vi "外观 1.vi"(0 "Data In":T5 caption="数据输入", 2 "Display State In":T3 caption="显示状态输入", 3 "Container State":T4 caption="容器状态") -> (6 "Data Out":T5 caption="数据输出", 7 "Display State Out":T3 caption="显示状态输出", 8 "Action":T2 caption="动作")   [LabVIEW 2016, in "曲线模型.xctl"]
uses:
  <vilib>/_xctls/Container State.ctl
  <vilib>/_xctls/Action.ctl
  <vilib>/_xctls/XControlSupport.lvlib
  <vilib>/Utility/config.llb/NI_LVConfig.lvlib
panel:
  in  "曲线模型":T1={"标液浓度1"=0.0, "样品1 F0"=0.0, "样品1 F1"=0.0, "测量吸光度1"=0.0, "样品1启用"=FALSE, "标液浓度2"=0.0, "样品2 F0"=0.0, "样品2 F1"=0.0, "测量吸光度2"=0.0, "样品2启用"=FALSE, "标液浓度3"=0.0, "样品3 F0"=0.0, "样品3 F1"=0.0, "测量吸光度3"=0.0, "样品3启用"=FALSE, "标液浓度4"=0.0, "样品4 F0"=0.0, "样品4 F1"=0.0, "测量吸光度4"=0.0, "样品4启用"=FALSE, "标液浓度5"=0.0, "样品5 F0"=0.0, "样品5 F1"=0.0, "测量吸光度5"=0.0, "样品5启用"=FALSE, "模型"=enum."线性", "method"=0, "精度"=4.0, "XY图"=[], "拟合公式"="", "r^2"=0.0} {"method" items=["最小二乘", "最小绝对残差", "Bisquare"]; "r^2" format="%.7g"}
  # "标液浓度"
  # "F0"
  # "F1"
  # "吸光值显示"
  # "样品一"
  # "辅\n助\n计\n算\n区"
  # "样品二"
  # "样品三"
  # "样品四"
  # "样品五"
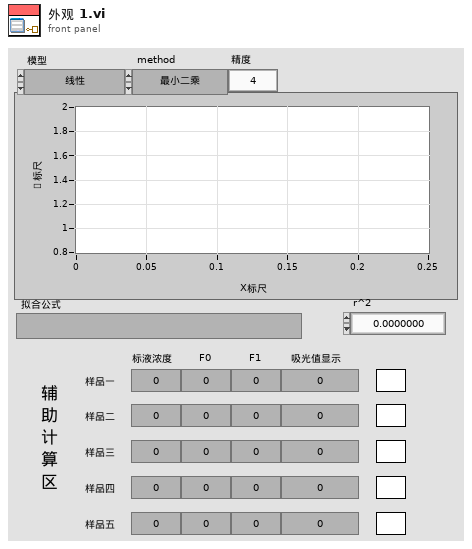
[diagram p1: front panel]
types:
  T1 = typedef "曲线模型.xctl/曲线模型外观.ctl" = cluster{"标液浓度1":dbl, "样品1 F0":dbl, "样品1 F1":dbl, "测量吸光度1":dbl, "样品1启用":bool, "标液浓度2":dbl, "样品2 F0":dbl, "样品2 F1":dbl, "测量吸光度2":dbl, "样品2启用":bool, "标液浓度3":dbl, "样品3 F0":dbl, "样品3 F1":dbl, "测量吸光度3":dbl, "样品3启用":bool, "标液浓度4":dbl, "样品4 F0":dbl, "样品4 F1":dbl, "测量吸光度4":dbl, "样品4启用":bool, "标液浓度5":dbl, "样品5 F0":dbl, "样品5 F1":dbl, "测量吸光度5":dbl, "样品5启用":bool, "模型":enum32{"线性", "多项式"}, "method":u16, "精度":dbl, "XY图":cluster{"X Values":dbl[], "Y Values":dbl[]}[], "拟合公式":string, "r^2":dbl}
  T2 = typedef "XControlSupport.lvlib/Action.ctl" = cluster{"Data Changed?":bool, "State Changed?":bool, "Action Name":string}
  T3 = typedef "曲线模型.xctl/状态 1.ctl" = cluster{"模型选择":cluster{"参数":u8, "测量模式":u8, "量程":u8}}
  T4 = typedef "XControlSupport.lvlib/Container State.ctl" = cluster{"Indicator?":bool, "Run Mode?":bool, " Refnum":refnum<vi>}
  T5 = typedef "曲线模型.xctl/数据 1.ctl" = cluster{"X^2":dbl, "X":dbl, "B":dbl}
  T6 = cluster{"曲线模型":cluster{"标液浓度1":dbl, "样品1 F0":dbl, "样品1 F1":dbl, "测量吸光度1":dbl, "样品1启用":bool, "标液浓度2":dbl, "样品2 F0":dbl, "样品2 F1":dbl, "测量吸光度2":dbl, "样品2启用":bool, "标液浓度3":dbl, "样品3 F0":dbl, "样品3 F1":dbl, "测量吸光度3":dbl, "样品3启用":bool, "标液浓度4":dbl, "样品4 F0":dbl, "样品4 F1":dbl, "测量吸光度4":dbl, "样品4启用":bool, "标液浓度5":dbl, "样品5 F0":dbl, "样品5 F1":dbl, "测量吸光度5":dbl, "样品5启用":bool, "模型":enum32{"线性", "多项式"}, "method":u16, "精度":dbl, "XY图":cluster{"X Values":dbl[], "Y Values":dbl[]}[], "拟合公式":string, "r^2":dbl}, "Polynomial Coefficients":dbl[]}
  T7 = typedef "NI_LVConfig.lvlib/Config Data RefNum.ctl" = refnum<k1>
  T8 = cluster{"Polynomial Coefficients[0]":dbl, "Polynomial Coefficients[1]":dbl, "Polynomial Coefficients[2]":dbl}
  T9 = cluster{"标液浓度1":dbl, "样品1 F0":dbl, "样品1 F1":dbl, "测量吸光度1":dbl, "样品1启用":bool, "标液浓度2":dbl, "样品2 F0":dbl, "样品2 F1":dbl, "测量吸光度2":dbl, "样品2启用":bool, "标液浓度3":dbl, "样品3 F0":dbl, "样品3 F1":dbl, "测量吸光度3":dbl, "样品3启用":bool, "标液浓度4":dbl, "样品4 F0":dbl, "样品4 F1":dbl, "测量吸光度4":dbl, "样品4启用":bool, "标液浓度5":dbl, "样品5 F0":dbl, "样品5 F1":dbl, "测量吸光度5":dbl, "样品5启用":bool, "模型":enum32{"线性", "多项式"}, "method":u16, "精度":dbl, "XY图":cluster{"X Values":dbl[], "Y Values":dbl[]}[], "拟合公式":string, "r^2":dbl}
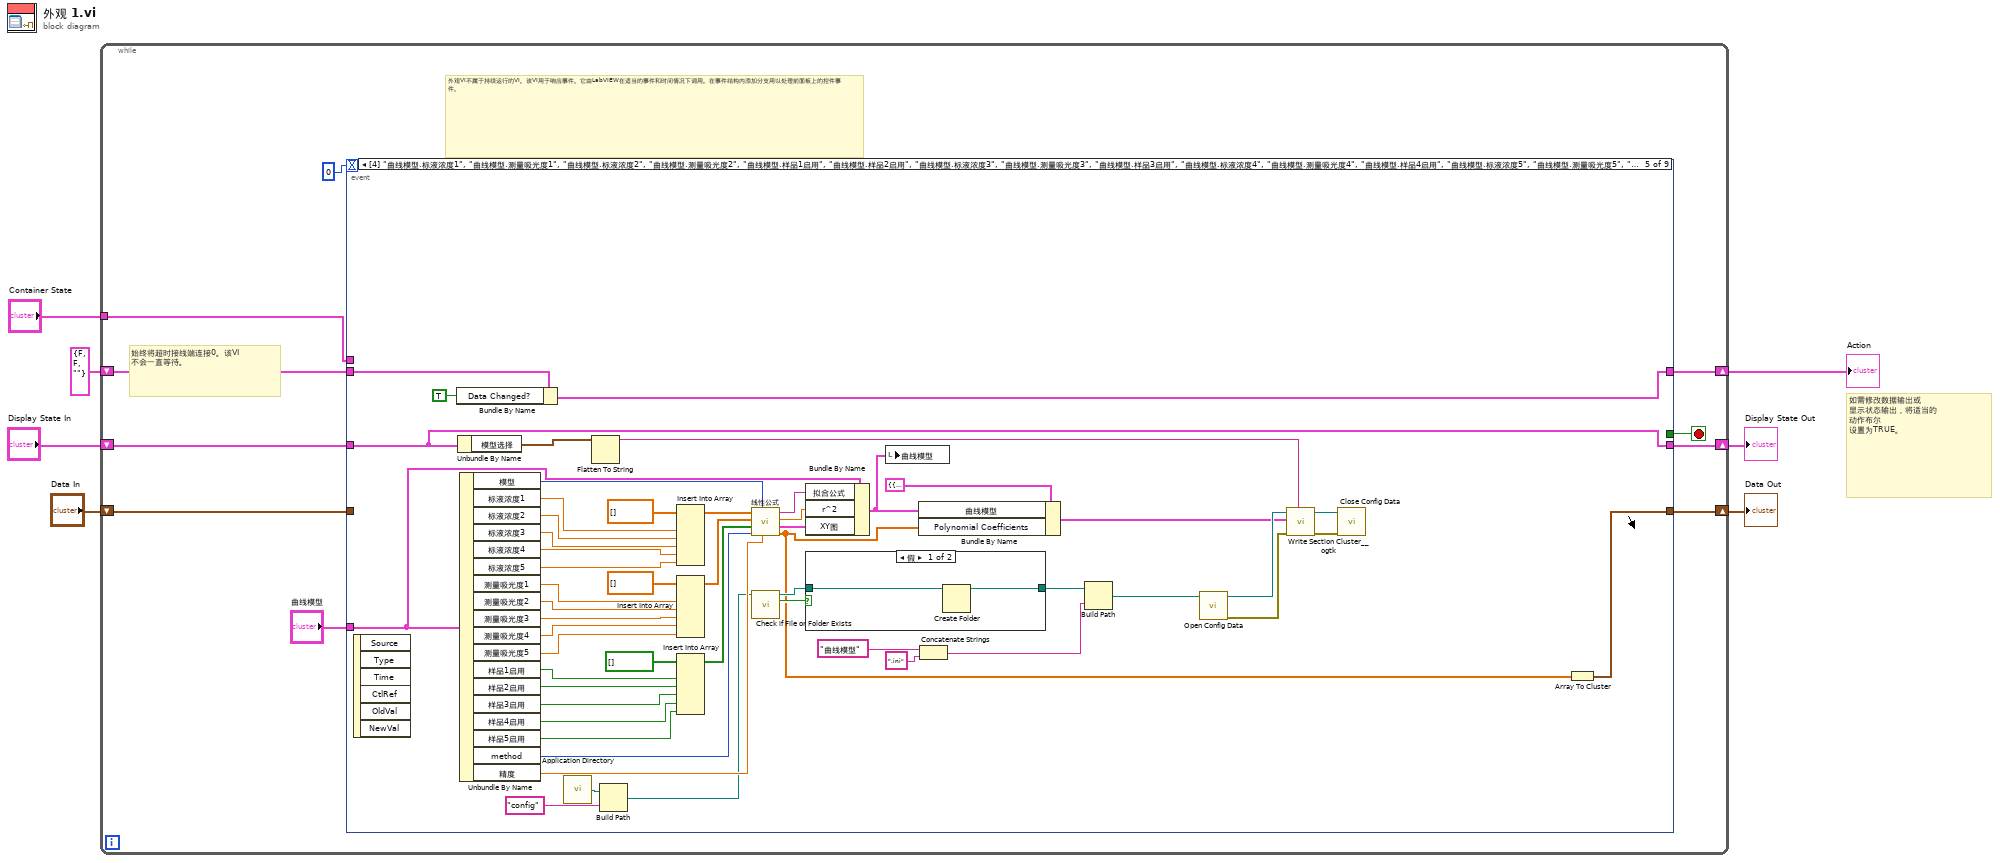
[diagram p0: block diagram]
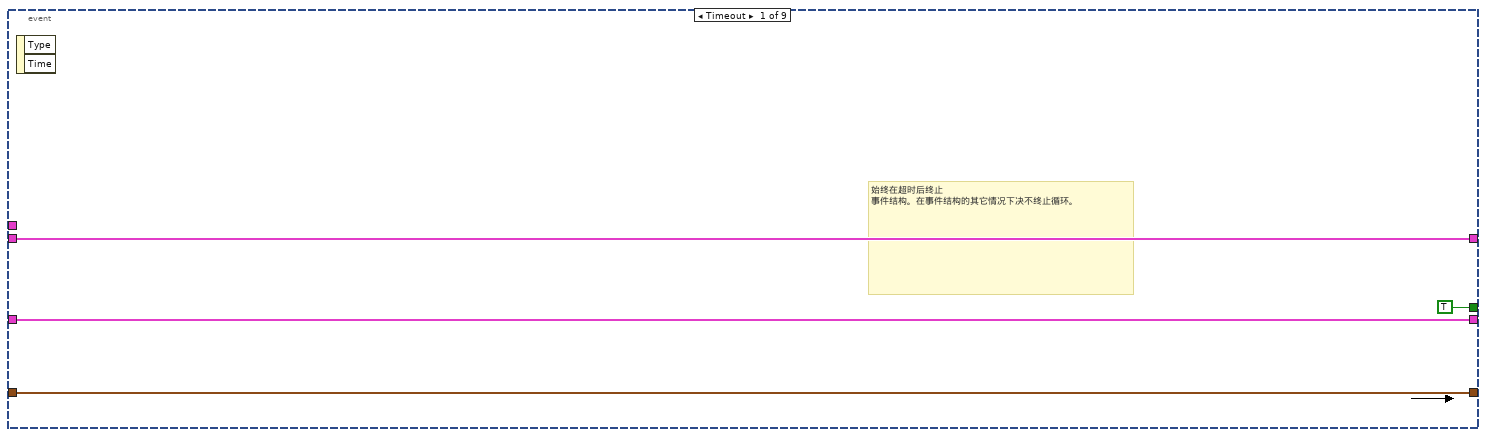
[diagram p2: hidden frame]
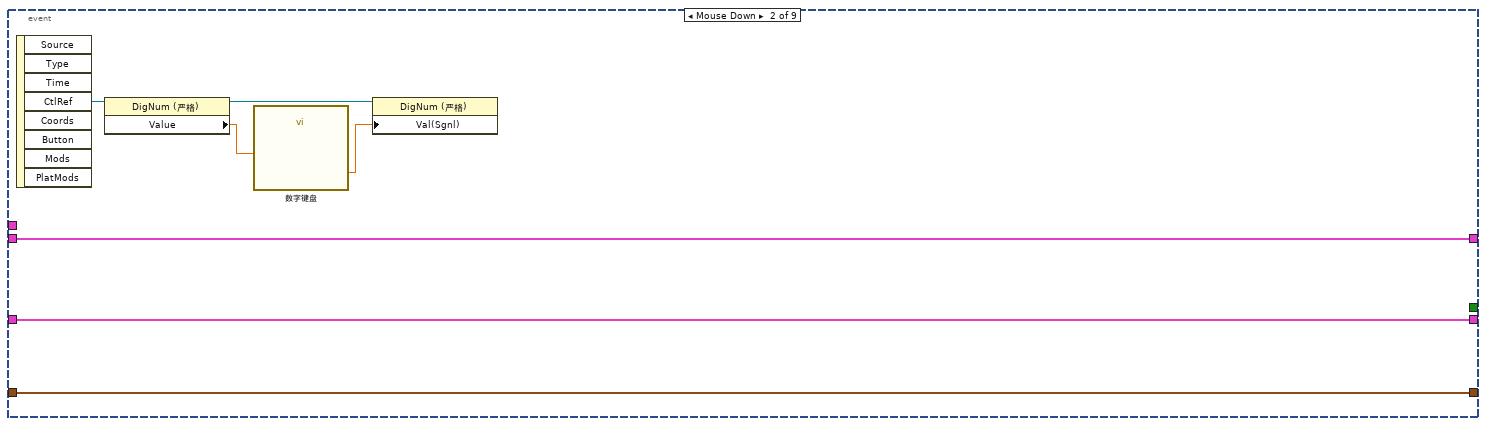
[diagram p3: hidden frame]
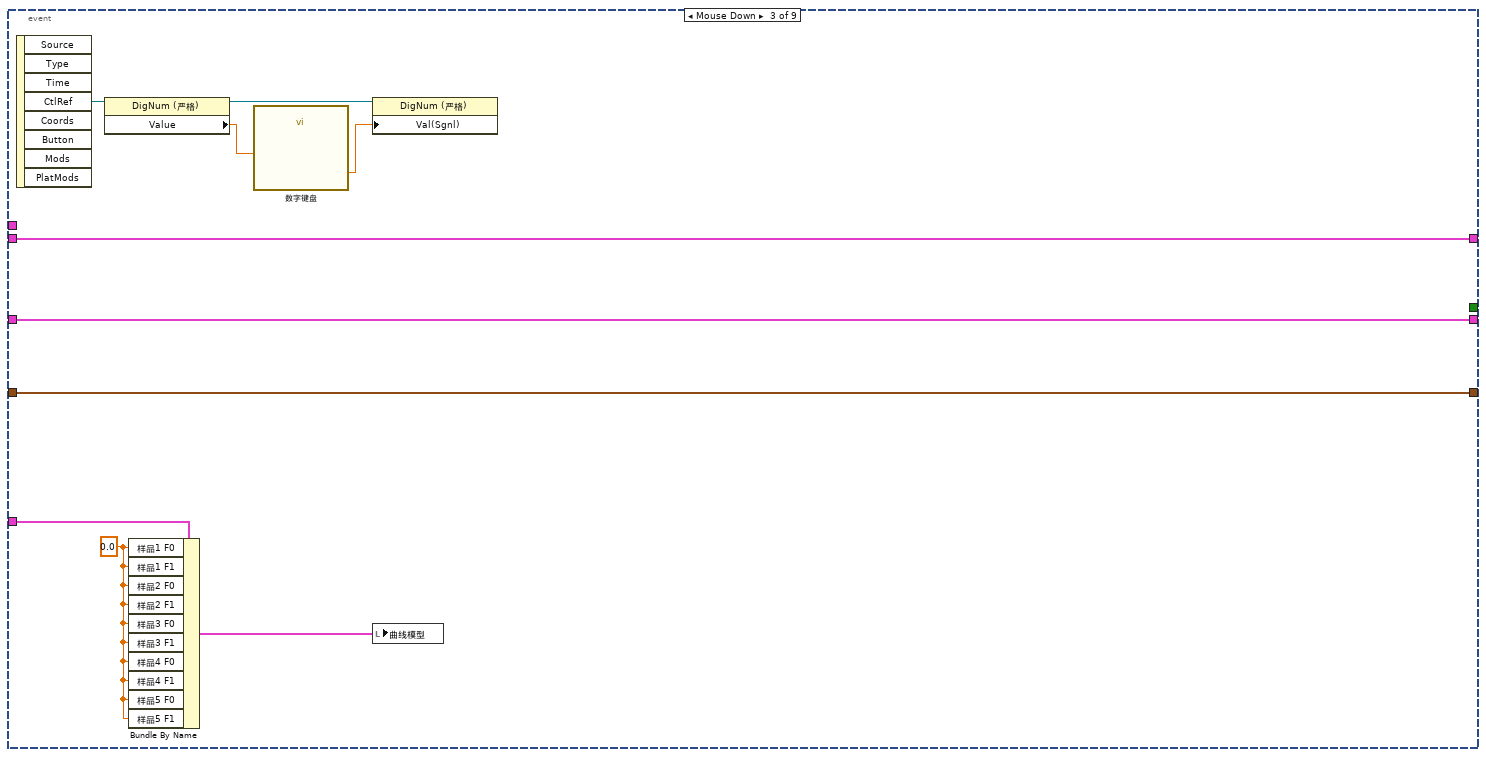
[diagram p4: hidden frame]
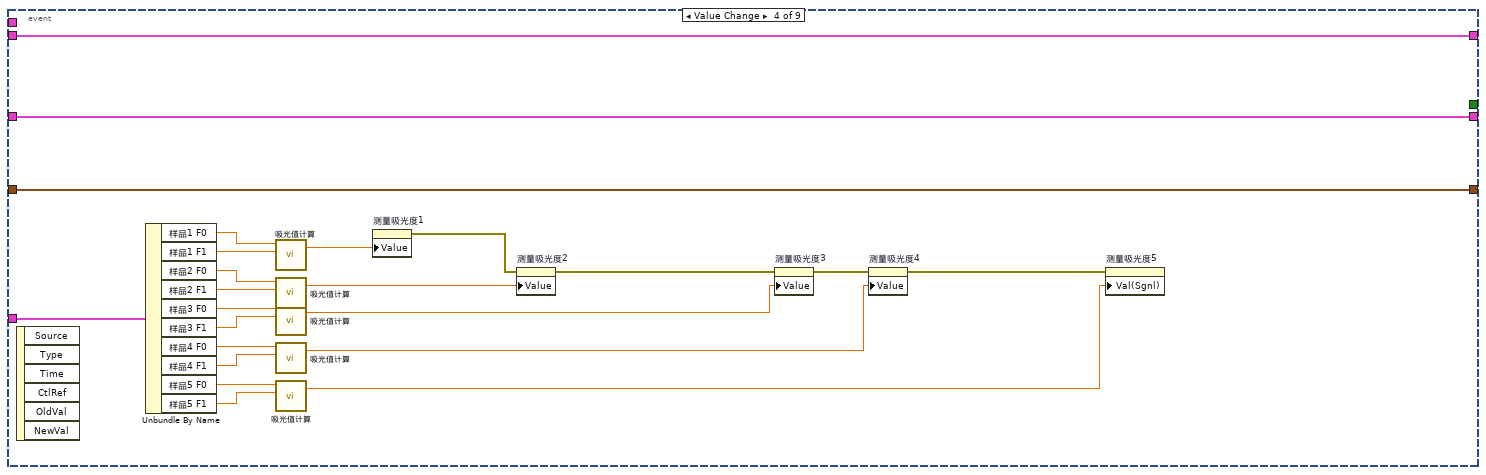
[diagram p5: hidden frame]
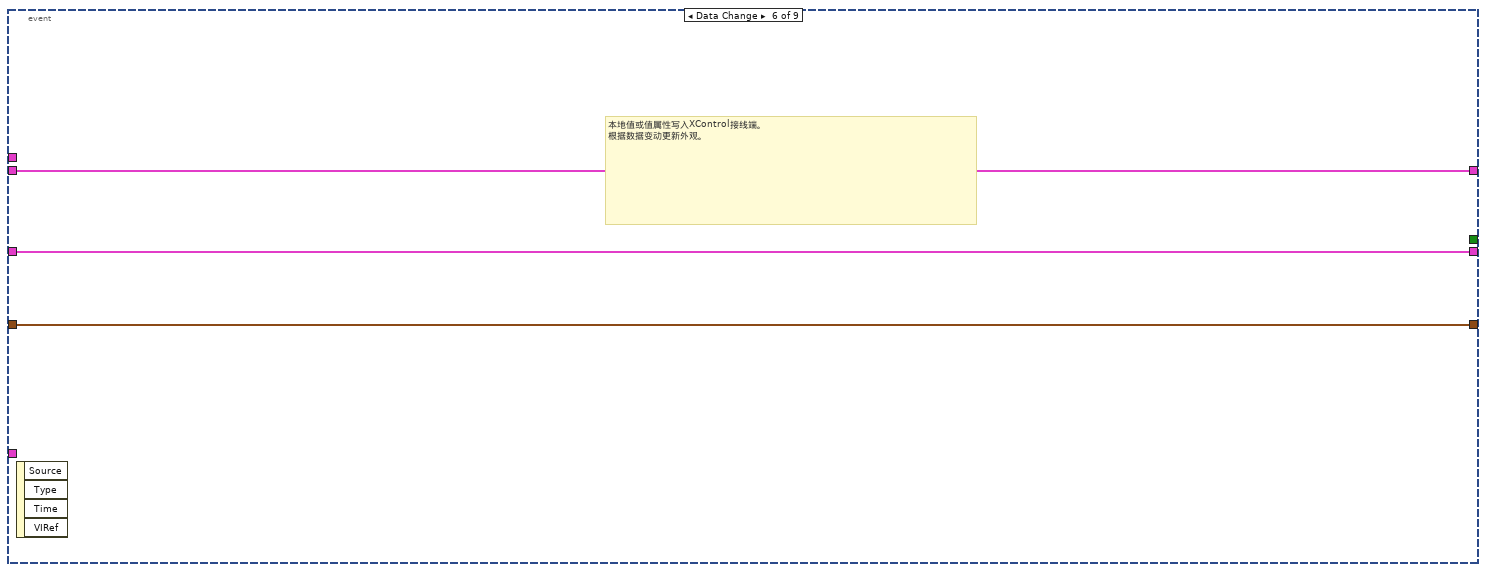
[diagram p7: hidden frame]
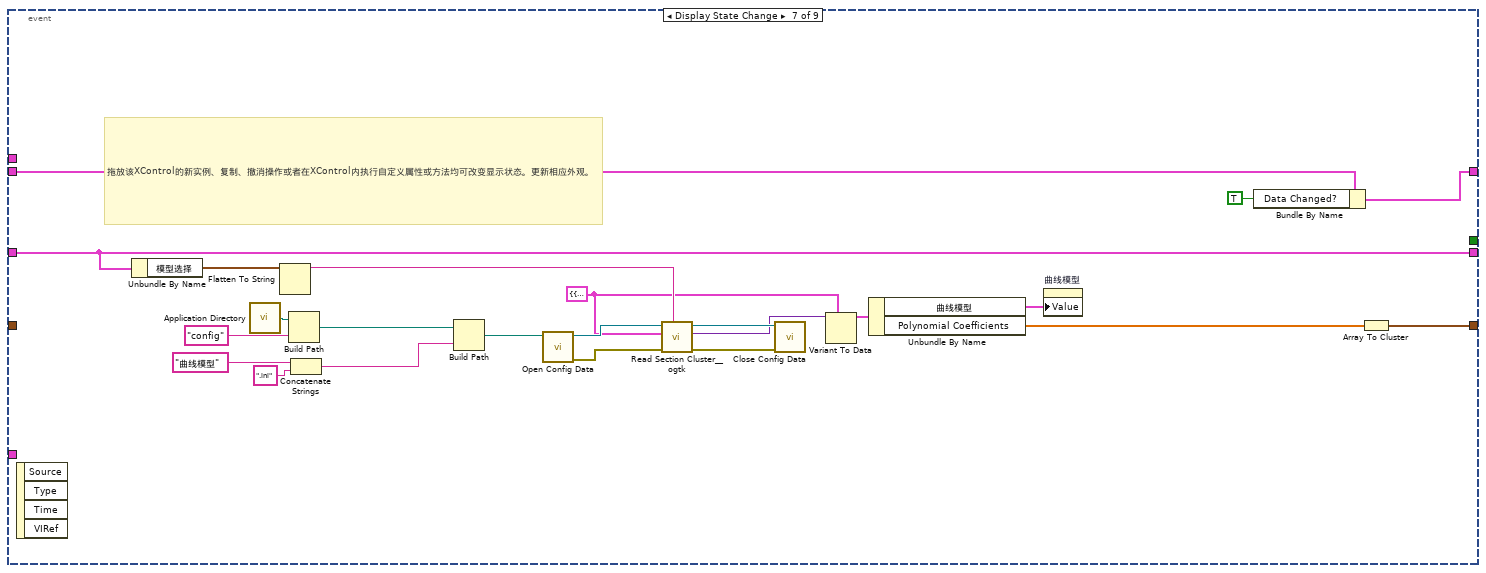
[diagram p8: hidden frame]
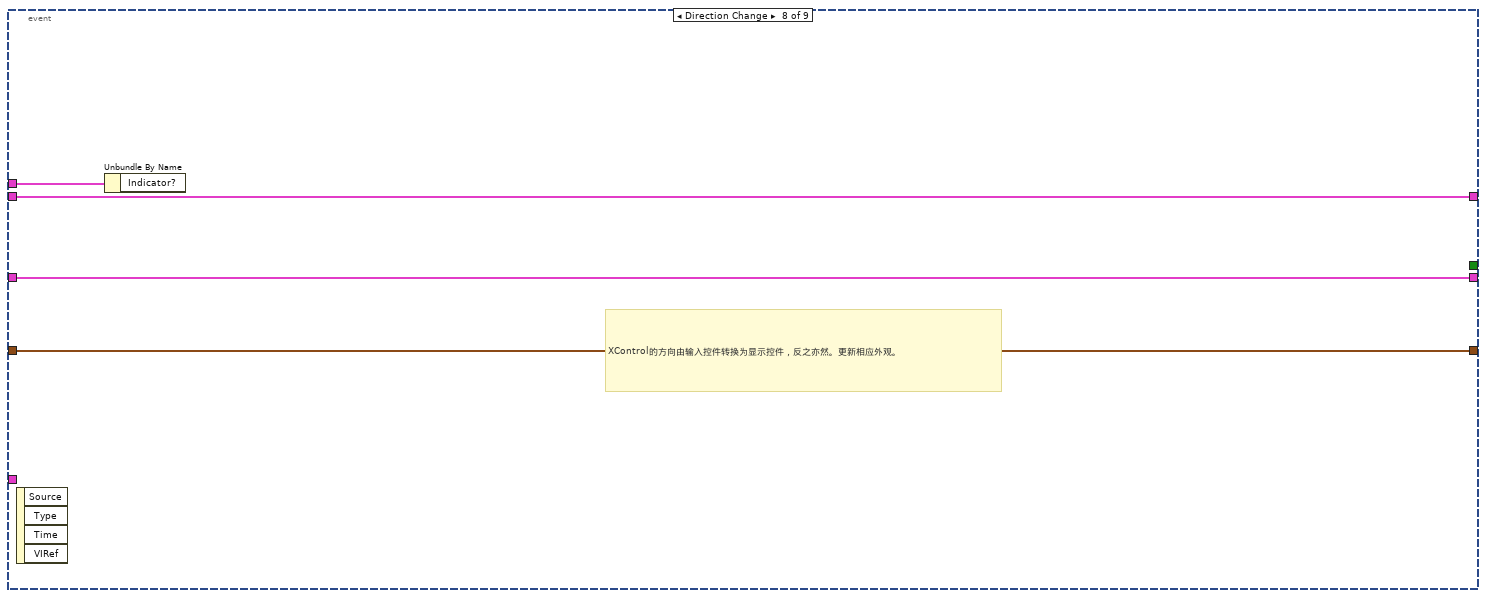
[diagram p9: hidden frame]
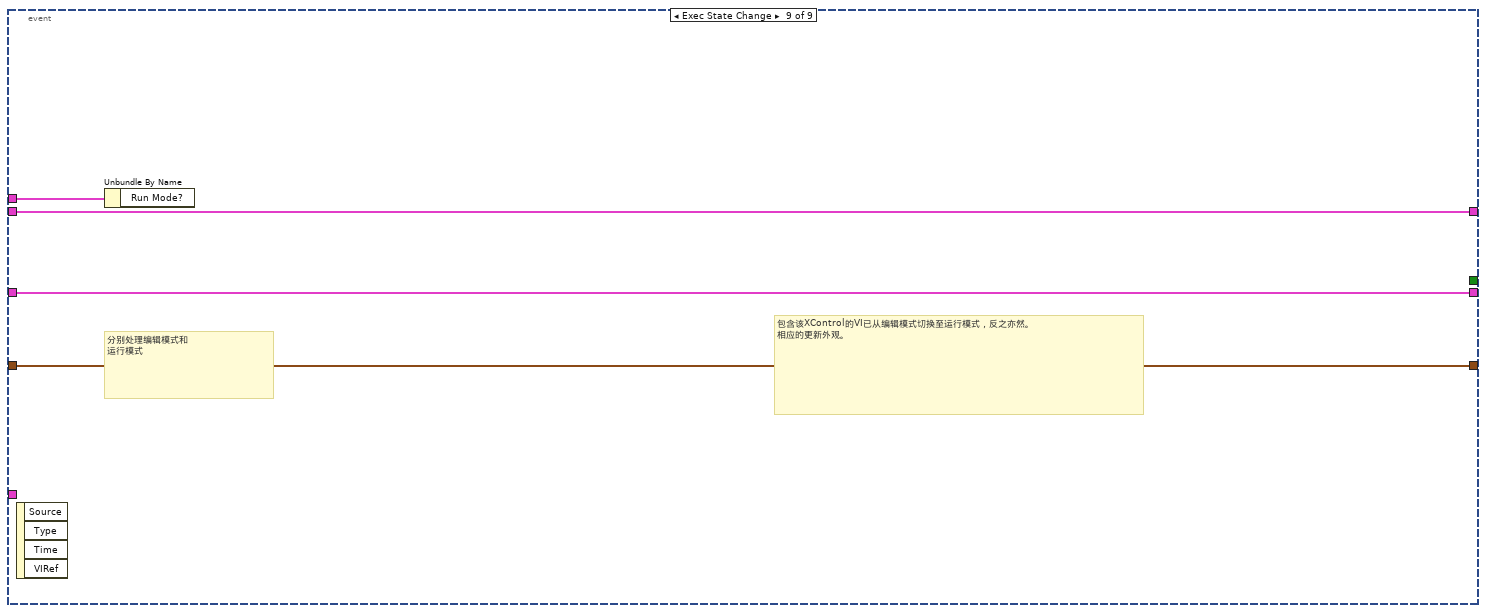
[diagram p10: hidden frame]
diagram:
  # "如需修改数据输出或\n显示状态输出，将适当的\n动作布尔\n设置为TRUE。"
  n1 = while {
    shift-right: [w16] -> w4
    shift-left: "Display State In" -> [w17]
    tunnel: "Container State" -> [w13]
    shift-right: [w11] -> w7
    shift-left: "Data In" -> [w12]
    shift-right: [w9] -> w2
    shift-left: T2 {"Data Changed?"=FALSE, "State Changed?"=FALSE, "Action Name"=""} ("Action") -> [w10]
    stop <- w15 stop-if-true
    # "外观VI不属于持续运行的VI。该VI用于响应事件。它由LabVIEW在适当的事件和时间情况下调用。在事件结构内添加分支用以处理前面板上的控件事件。"
    # "始终将超时接线端连接0。该VI\n不会一直等待。"
    n2 = event shown="[4] \"曲线模型.标液浓度1\", \"曲线模型.测量吸光度1\", \"曲线模型.标液浓度2\", \"曲线模型.测量吸光度2\", \"曲线模型.样品1启用\", \"曲线模型.样品2启用\", \"曲线模型.标液浓度3\", \"曲线模型.测量吸光度3\", \"曲线模型.样品3启用\", \"曲线模型.标液浓度4\", \"曲线模型.测量吸光度4\", \"曲线模型.样品4启用\", \"曲线模型.标液浓度5\", \"曲线模型.测量吸光度5\", \"曲线模型.样品5启用\", \"曲线模型.模型\", \"曲线模型.method\", \"曲线模型.精度\": 值改变" {
      selector: _ -> [_ _ _ _ _ _ _ _ _]
      dyn-events: _ -> [_ _ _ _ _ _ _ _ _]
      timeout: 0 -> [_ _ _ _ _ _ _ _ _]
      tunnel: w17 -> [w19 w28 w38 w61 w74 w118 w138 w146 w150]
      tunnel: [w19 w28 w38 w61 w74 w118 w138 w146 w150] -> w16
      tunnel: [TRUE _ _ _ _ _ _ _ _] -> w15
      tunnel: w13 -> [_ _ _ _ _ _ _ w147 w151]
      tunnel: w12 -> [w18 w27 w37 w60 _ w120 _ w145 w149]
      tunnel: [w18 w27 w37 w60 w86 w120 w124 w145 w149] -> w11
      tunnel: [w20 w26 w36 w59 w83 w119 w121 w144 w148] -> w9
      tunnel: w10 -> [w20 w26 w36 w59 w85 w119 w123 w144 w148]
      tunnel: "曲线模型" -> [_ _ w31 w48 w90 _ _ _ _]
      event Timeout {
        # "始终在超时后终止\n事件结构。在事件结构的其它情况下决不终止循环。"
        n3 = event-data() -> ()  [unwired: 1 in, 2 out]
      }
      event Mouse Down {
        n4 = event-data() -> ("CtlRef"=w25:refnum<vi>)  [unwired: 1 in, 7 out]
        n5 = property class="DigNum (严格)"(reference=w25) -> (reference out=w22:refnum<vi>, "Value"=w24:dbl)  [unwired: 1 in, 1 out]
        n6 = call "数字键盘.vi"("OldNumber"=w24) -> ("NewNumber"=w23:dbl)
        n7 = property class="DigNum (严格)"(reference=w22, "Val(Sgnl)"=w23) -> ()  [unwired: 1 in, 2 out]
      }
      event Mouse Down {
        w30 = 0.0 ("测量吸光度1")
        n8 = event-data() -> ("CtlRef"=w35:refnum<vi>)  [unwired: 1 in, 7 out]
        n9 = property class="DigNum (严格)"(reference=w35) -> (reference out=w32:refnum<vi>, "Value"=w34:dbl)  [unwired: 1 in, 1 out]
        n10 = Bundle By Name(cluster=w31, "样品1 F0"=w30, "样品1 F1"=w30, "样品2 F0"=w30, "样品2 F1"=w30, "样品3 F0"=w30, "样品3 F1"=w30, "样品4 F0"=w30, "样品4 F1"=w30, "样品5 F0"=w30, "样品5 F1"=w30) -> (w29:T1)
        n11 = call "数字键盘.vi"("OldNumber"=w34) -> ("NewNumber"=w33:dbl)
        n12 = property class="DigNum (严格)"(reference=w32, "Val(Sgnl)"=w33) -> ()  [unwired: 1 in, 2 out]
        n13 = local write "曲线模型"(w29) -> ()
      }
      event Value Change {
        n14 = event-data() -> ()  [unwired: 1 in, 6 out]
        n15 = Unbundle By Name(w48) -> ("样品1 F0"=w58:dbl, "样品1 F1"=w57:dbl, "样品2 F0"=w49:dbl, "样品2 F1"=w50:dbl, "样品3 F0"=w51:dbl, "样品3 F1"=w52:dbl, "样品4 F0"=w53:dbl, "样品4 F1"=w54:dbl, "样品5 F0"=w55:dbl, "样品5 F1"=w56:dbl)
        n16 = call "吸光值计算.vi"("F1"=w57, "F0"=w58) -> ("测量吸光度"=w43:dbl)  [unwired: 3 in]
        n17 = call "吸光值计算.vi"("F1"=w50, "F0"=w49) -> ("测量吸光度"=w42:dbl)  [unwired: 3 in]
        n18 = call "吸光值计算.vi"("F1"=w52, "F0"=w51) -> ("测量吸光度"=w41:dbl)  [unwired: 3 in]
        n19 = call "吸光值计算.vi"("F1"=w54, "F0"=w53) -> ("测量吸光度"=w40:dbl)  [unwired: 3 in]
        n20 = call "吸光值计算.vi"("F1"=w56, "F0"=w55) -> ("测量吸光度"=w39:dbl)  [unwired: 3 in]
        n21 = property on="测量吸光度1" class="DigNum (严格)"("Value"=w43) -> (error out=w47:errorcluster)  [unwired: 2 in, 1 out]
        n22 = property on="测量吸光度2" class="DigNum (严格)"(error in=w47, "Value"=w42) -> (error out=w46:errorcluster)  [unwired: 1 in, 1 out]
        n23 = property on="测量吸光度3" class="DigNum (严格)"(error in=w46, "Value"=w41) -> (error out=w45:errorcluster)  [unwired: 1 in, 1 out]
        n24 = property on="测量吸光度4" class="DigNum (严格)"(error in=w45, "Value"=w40) -> (error out=w44:errorcluster)  [unwired: 1 in, 1 out]
        n25 = property on="测量吸光度5" class="DigNum (严格)"(error in=w44, "Val(Sgnl)"=w39) -> ()  [unwired: 1 in, 2 out]
      }
      event Value Change {
        n26 = event-data() -> ()  [unwired: 1 in, 6 out]
        n27 = Bundle By Name(cluster=w85, "Data Changed?"=TRUE) -> (w83:T2)
        n28 = Unbundle By Name(w74) -> ("模型选择"=w73:cluster{"参数":u8, "测量模式":u8, "量程":u8})
        n29 = Unbundle By Name(w90) -> ("模型"=w114:enum32{"线性", "多项式"}, "标液浓度1"=w110:dbl, "标液浓度2"=w109:dbl, "标液浓度3"=w108:dbl, "标液浓度4"=w107:dbl, "标液浓度5"=w106:dbl, "测量吸光度1"=w103:dbl, "测量吸光度2"=w102:dbl, "测量吸光度3"=w101:dbl, "测量吸光度4"=w100:dbl, "测量吸光度5"=w99:dbl, "样品1启用"=w96:bool, "样品2启用"=w95:bool, "样品3启用"=w94:bool, "样品4启用"=w93:bool, "样品5启用"=w92:bool, "method"=w113:u16, "精度"=w112:dbl)
        n30 = call <vilib>:"Application Directory.vi"() -> ("Application Directory"=w82:path)
        n31 = Flatten To String(anything=w73) -> (data string=w72:string)  [unwired: 3 in, 2 out]
        n32 = Build Path(base path=w82, name or relative path="config" ("名称或相对路径")) -> (appended path=w80:path)
        n33 = Insert Into Array(array=dbl[] [] ("标液浓度"), new element #1=w110, new element #2=w109, new element #3=w108, new element #4=w107, new element #5=w106) -> (w105:dbl[])  [unwired: 1 in]
        n34 = Insert Into Array(array=dbl[] [] ("标液浓度"), new element #1=w103, new element #2=w102, new element #3=w101, new element #4=w100, new element #5=w99) -> (w98:dbl[])  [unwired: 1 in]
        n35 = Insert Into Array(array=bool[] [] ("启用"), new element #1=w96, new element #2=w95, new element #3=w94, new element #4=w93, new element #5=w92) -> (w91:bool[])  [unwired: 1 in]
        n36 = call "线性公式.vi"("精度"=w112, "模型"=w114, "method"=w113, "启用"=w91, "监测浓度"=w98, "标液浓度"=w105) -> ("Polynomial Coefficients"=w63:dbl[], "XY图"=w87:cluster{"X Values":dbl[], "Y Values":dbl[]}[], "r^2"=w88:dbl, "拟合方程"=w89:string)  [unwired: 2 in]
        n37 = call <vilib>:"Check if File or Folder Exists.vi"("path"=w80) -> ("file or folder exists?"=w79:bool, "dup path"=w78:path)  [unwired: 8 in, 1 out]
        n38 = Bundle By Name(cluster=w90, "拟合公式"=w89, "r^2"=w88, "XY图"=w87) -> (w64:T1)
        n39 = case shown="假" w79 {
          tunnel: w78 -> [w116 w117]
          tunnel: [w115 w117] -> w75
          frame False {
            n40 = Create Folder(path (use dialog)=w116) -> (created path=w115:path)  [unwired: 2 in, 2 out]
          }
          frame True {
          }
        }
        n41 = local write "曲线模型"(w64) -> ()
        n42 = Bundle By Name(cluster=T6 {"曲线模型"={"标液浓度1"=0.0, "样品1 F0"=0.0, "样品1 F1"=0.0, "测量吸光度1"=0.0, "样品1启用"=FALSE, "标液浓度2"=0.0, "样品2 F0"=0.0, "样品2 F1"=0.0, "测量吸光度2"=0.0, "样品2启用"=FALSE, "标液浓度3"=0.0, "样品3 F0"=0.0, "样品3 F1"=0.0, "测量吸光度3"=0.0, "样品3启用"=FALSE, "标液浓度4"=0.0, "样品4 F0"=0.0, "样品4 F1"=0.0, "测量吸光度4"=0.0, "样品4启用"=FALSE, "标液浓度5"=0.0, "样品5 F0"=0.0, "样品5 F1"=0.0, "测量吸光度5"=0.0, "样品5启用"=FALSE, "模型"=enum."线性", "method"=0, "精度"=4.0, "XY图"=[], "拟合公式"="", "r^2"=0.0}, "Polynomial Coefficients"=[]} ("输出簇"), "曲线模型"=w64, "Polynomial Coefficients"=w63) -> (w62:T6)
        n43 = Concatenate Strings("曲线模型" ("字符串"), ".ini" ("字符串")) -> (w77:string)
        n44 = Build Path(base path=w75, name or relative path=w77) -> (appended path=w66:path)
        n45 = call <vilib>:"Open Config Data.vi"("configuration file path"=w66) -> ("error out"=w69:errorcluster, "refnum"=w70:T7)  [unwired: 8 in, 1 out]
        n46 = call <userlib>:"Write Section Cluster__ogtk.vi"("section (optional)"=w72, "error in (no error)"=w69, "Section Formatted Cluster"=w62, "refnum"=w70) -> ("error out"=w67:errorcluster, "dup refnum"=w68:T7)  [unwired: 6 in]
        n47 = call <vilib>:"Close Config Data.vi"("error in (no error)"=w67, "refnum"=w68) -> ()  [unwired: 8 in, 2 out]
        n48 = Array To Cluster(array=w63) -> (cluster=w86:T8)
      }
      event Data Change {
        # "本地值或值属性写入XControl接线端。\n根据数据变动更新外观。"
        n49 = event-data() -> ()  [unwired: 1 in, 4 out]
      }
      event Display State Change {
        w128 = T6 {"曲线模型"={"标液浓度1"=0.0, "样品1 F0"=0.0, "样品1 F1"=0.0, "测量吸光度1"=0.0, "样品1启用"=FALSE, "标液浓度2"=0.0, "样品2 F0"=0.0, "样品2 F1"=0.0, "测量吸光度2"=0.0, "样品2启用"=FALSE, "标液浓度3"=0.0, "样品3 F0"=0.0, "样品3 F1"=0.0, "测量吸光度3"=0.0, "样品3启用"=FALSE, "标液浓度4"=0.0, "样品4 F0"=0.0, "样品4 F1"=0.0, "测量吸光度4"=0.0, "样品4启用"=FALSE, "标液浓度5"=0.0, "样品5 F0"=0.0, "样品5 F1"=0.0, "测量吸光度5"=0.0, "样品5启用"=FALSE, "模型"=enum."线性", "method"=0, "精度"=4.0, "XY图"=[], "拟合公式"="", "r^2"=0.0}, "Polynomial Coefficients"=[]} ("输出簇")
        # "拖放该XControl的新实例、复制、撤消操作或者在XControl内执行自定义属性或方法均可改变显示状态。更新相应外观。"
        n50 = event-data() -> ()  [unwired: 1 in, 4 out]
        n51 = Unbundle By Name(w138) -> ("模型选择"=w131:cluster{"参数":u8, "测量模式":u8, "量程":u8})
        n52 = call <vilib>:"Application Directory.vi"() -> ("Application Directory"=w137:path)
        n53 = Flatten To String(anything=w131) -> (data string=w130:string)  [unwired: 3 in, 2 out]
        n54 = Build Path(base path=w137, name or relative path="config" ("名称或相对路径")) -> (appended path=w135:path)
        n55 = Concatenate Strings("曲线模型" ("字符串"), ".ini" ("字符串")) -> (w133:string)
        n56 = Build Path(base path=w135, name or relative path=w133) -> (appended path=w139:path)
        n57 = call <vilib>:"Open Config Data.vi"("configuration file path"=w139) -> ("error out"=w142:errorcluster, "refnum"=w143:T7)  [unwired: 8 in, 1 out]
        n58 = call <userlib>:"Read Section Cluster__ogtk.vi"("section (optional)"=w130, "error in (no error)"=w142, "Section Formatted Cluster Type"=w128, "refnum"=w143) -> ("error out"=w140:errorcluster, "Section Formatted Cluster"=w132:variant, "dup refnum"=w141:T7)  [unwired: 3 in, 2 out]
        n59 = call <vilib>:"Close Config Data.vi"("error in (no error)"=w140, "refnum"=w141) -> ()  [unwired: 8 in, 2 out]
        n60 = Variant To Data(type=w128, Variant=w132) -> (data=w127:T6)  [unwired: 1 in, 1 out]
        n61 = Unbundle By Name(w127) -> ("曲线模型"=w126:T9, "Polynomial Coefficients"=w125:dbl[])
        n62 = property on="曲线模型" class="Clust (严格)"("Value"=w126) -> ()  [unwired: 2 in, 2 out]
        n63 = Bundle By Name(cluster=w123, "Data Changed?"=TRUE) -> (w121:T2)
        n64 = Array To Cluster(array=w125) -> (cluster=w124:T8)
      }
      event Direction Change {
        # "XControl的方向由输入控件转换为显示控件，反之亦然。更新相应外观。"
        n65 = event-data() -> ()  [unwired: 1 in, 4 out]
        n66 = Unbundle By Name(w147) -> ()  [unwired: 1 out]
      }
      event Exec State Change {
        # "包含该XControl的VI已从编辑模式切换至运行模式，反之亦然。\n相应的更新外观。"
        # "分别处理编辑模式和\n运行模式"
        n67 = event-data() -> ()  [unwired: 1 in, 4 out]
        n68 = Unbundle By Name(w151) -> ()  [unwired: 1 out]
      }
    }
  }
  "Display State Out" <- w4
  "Data Out" <- w7
  "Action" <- w2
